vi "Method Quack.vi"(0 "Duck in":refnum<class "Duck.lvclass">, 11 "error in (no error)":errorcluster) -> (4 "Duck out":refnum<class "Duck.lvclass">, 15 "error out":errorcluster)   [LabVIEW 2021, in "Duck.lvclass"]
uses:
  Duck.lvclass
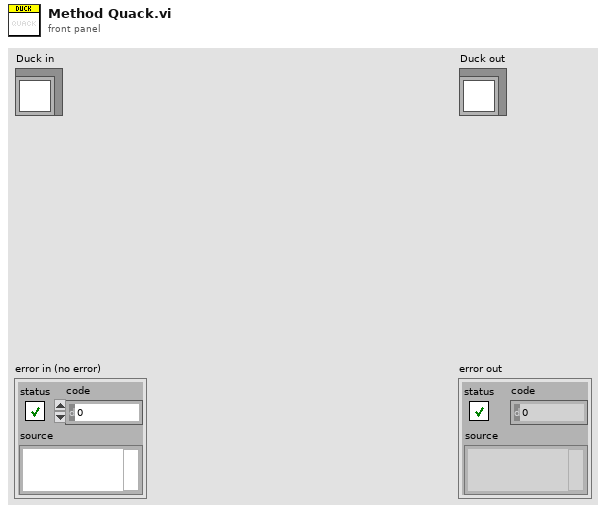
[diagram p1: front panel]
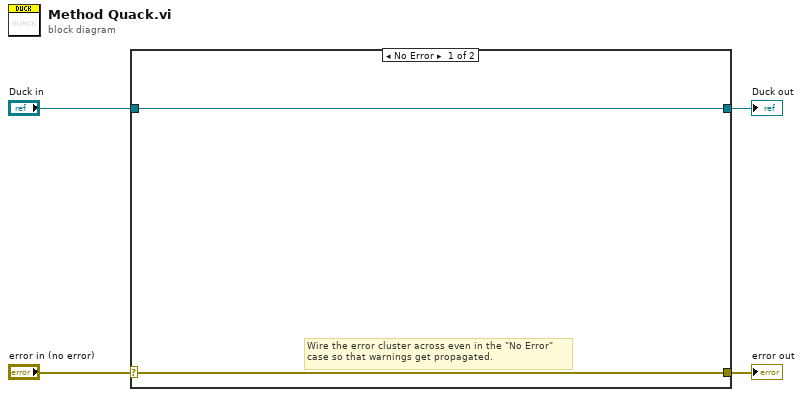
[diagram p0: block diagram]
diagram:
  n1 = case shown="No Error" "error in (no error)" {
    selector: "error in (no error)" -> [w5 w8]
    tunnel: [w5 w8] -> w3
    tunnel: [w6 w7] -> w1
    tunnel: "Duck in" -> [w6 w7]
    frame No Error {
      # "Wire the error cluster across even in the \"No Error\"\ncase so that warnings get propagated."
    }
    frame Error {
    }
  }
  "error out" <- w3
  "Duck out" <- w1
